vi "read raw default value.vi"(8 "error in":errorcluster, 11 "system tag in":refnum<class "data bus tag description.lvclass">) -> (0 "error out":errorcluster, 2 "raw default":variant, 3 "system tag out":refnum<class "data bus tag description.lvclass">)   [LabVIEW 2013, in "data bus tag description.lvclass"]
doc: "Reads the default value field stored in the tag descriptor. This is returned as a raw string, not as an interpreted data type."
uses:
  data bus tag description.lvclass
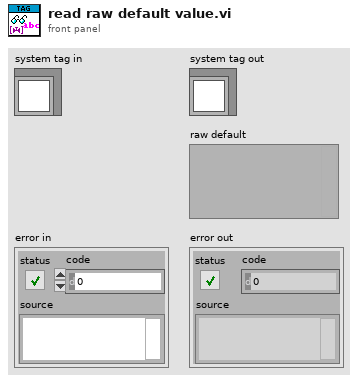
[diagram p1: front panel]
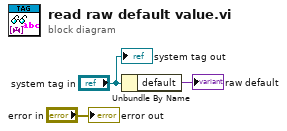
[diagram p0: block diagram]
diagram:
  n1 = Unbundle By Name("system tag in") -> ("default"=→"raw default":variant)
  "system tag out" <- "system tag in"
  "error out" <- "error in"
